vi "LET Transfer v1.vi"() -> ()   [LabVIEW 2010]
doc: "Cont(inuous) Acq(uire) & Chart (hw timed) demonstrates the hardware timed, non-buffered technique of data acquisition. The scan clock on the board controls acquisition timing. Acquired scans are read directly from the device's FIFO using AI Single Scan. \n\nThe acquisition is configured with no buffer, and the on-board scan clock started at the selected scan rate. In the first loop iteration, the newest (most recent) scan is read from the FIFO. In each subsequent loop iteration AI Single Scan is called to read the oldest scan from the FIFO. Then if a scan is missed because the acquisition does not keep up, an error message will be displayed, and the acquisition stopped. Each scan is plotted on the chart after it is read. \n\nA common reason to use non-buffered acquisition is that some kind of processing needs to be done for each data point. You will probably want to add more functions to the diagram to customize this VI for your application. The acquisition rate you can achieve depends on how much processing and display the VI must do. This VI calls a subVI named My Single-Scan Processing. Add whatever processing you need to this subVI, or replace it with one of your own. The data processing subVI also demonstrates how to use error clusters in your own subVIs, so they can be included in the error data flow chain.\n\nBefore running this VI, set the values of the controls on the front panel. Select Show Help Window from the Help menu to see a description of each control. If the values you select for all the controls are values you will usually use, select Make Current Values Default from the Operate menu and save the VI. Or, you may save individual control's default values by popping up on the control, selecting Data Operations, then selecting Make Current Value Default, and saving the VI."
uses:
  <instrlib>/agilent_b2900_series/Agilent B2900 Series/Public/Configure/Measurement/Configure Measurement (Current).vi
  <instrlib>/agilent_b2900_series/Agilent B2900 Series/Public/Configure/Measurement/Configure Measurement (Voltage).vi
  <vilib>/Utility/file.llb/Write To Spreadsheet File (DBL).vi
  <instrlib>/agilent_b2900_series/Agilent B2900 Series/Agilent B2900 Series.lvlib
panel:
  out "Igs array 2":dbl[][](array[numeric])
  out "Vgs array 2":dbl[][](array[numeric])
  out "Vds array 2":dbl[][](array[numeric])
  out "Corrected PD current array 2":dbl[][](array[numeric])
  out "Ids array 2":dbl[][](array[numeric])
  out "corrected PD current array":dbl[](array[numeric])
  out "Vds array":dbl[](array[numeric])
  out "Ids array":dbl[](array[numeric])
  out "Vgs array":dbl[](array[numeric])
  out "Igs array":dbl[](array[numeric])
  in  "Tab Control":T1(tab)
  in  "keithley address":string="GPIB0::20::INSTR"
  in  "agilent address":refnum<visa-resource-name>="GPIB0::23::INSTR"
  in  "Initial Vgs (V)":sgl format="%.2f"
  in  "Vgs step (V)":sgl=1.0 format="%.2f"
  in  "Vgs delay time (ms)":sgl=10.0 format="%.2f"
  in  "Vgs delay after first value":sgl=10.0 caption="Vgs delay after first value (ms)" format="%.2f"
  in  "Final Vgs(V)":sgl=60.0 format="%.2f"
  in  "light emission ON/OFF":bool=TRUE
  in  "Vds step (V)":sgl=20.0 format="%.2f"
  in  "Final Vds (V)":sgl=60.0 format="%.2f"
  in  "Initial Vds (V)":sgl format="%.2f"
  in  "Vds hold time (ms)":i32=10
  in  "Compliance Voltage (channel 1)":dbl=60.0
  in  "Compliance Current (channel 2)":dbl=0.001
  in  "Compliance Voltage (channel 2)":dbl=60.0
  in  "Compliance Current (channel 1)":dbl=0.0001
  in  "keithley compliance limit":dbl(ring)=0.025 items=["25uA"=2.5e-05, "250uA"=0.00025, "2.5mA"=0.0025, "25mA"=0.025]
  in  "Loop":bool=TRUE
  in  "Tab Control 2":enum32{"log scale", "linear scale"}(tab)
  out "Current Scan log":cluster{dbl[], dbl[]}(graph) caption="Current Scan"
  out "Current Scan log2":cluster{dbl[], dbl[]}(graph) caption="Current Scan"
  out "Current Scan linear":cluster{dbl[], dbl[]}(graph) caption="Current Scan"
  out "Current Scan linear 2":cluster{dbl[], dbl[]}(graph) caption="Current Scan"
  out "Applied Vgs":sgl caption="current VDS (V)" format="%.2f"
  out "Applied Vds":sgl caption="current VDS (V)" format="%.2f"
  out "Measured Ids":dbl format="%.2e"
  out "Measured Vds":dbl
  out "corrected PD current":dbl format="%^.2e"
  out "dark PD current (A)":dbl format="%^.2e"
  out "PD current":dbl format="%^.2e"
  out "Measured Igs":dbl
  out "Measured Vgs":dbl
  out "channel 2 status":bool
  out "channel 1 status":bool
  out "half  points":sgl
  out "Vgs points":sgl
  out "Vds points":sgl
  in  "Tab Control 3":enum32{"Log scale", "Linear scale"}(tab)
  out "?":cluster{dbl[], dbl[]}[](graph)
  out "?":cluster{dbl[], dbl[]}[](graph)
  out "?":cluster{dbl[], dbl[]}[](graph)
  out "?":cluster{dbl[], dbl[]}[](graph)
  in  "error in keithley":errorcluster
  out "keithley address out":refnum<k15>
  out "error out keithley":errorcluster
  out "error out agilent":errorcluster
  out "Agilent address out":refnum<visa-resource-name>
  # "LET Transfer v1"
  # "Gate Setting"
  # "Drain-source Setting"
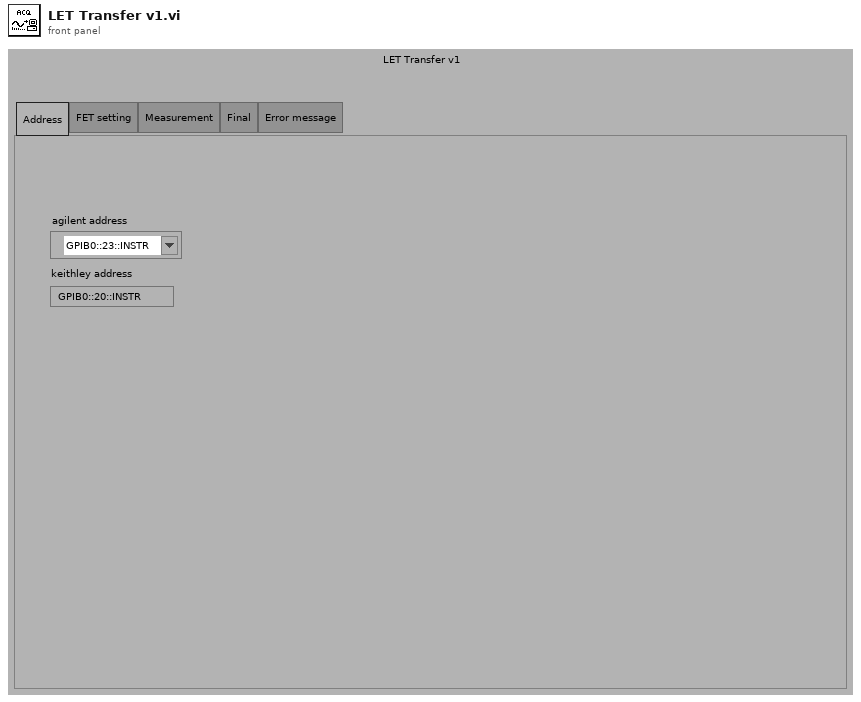
[diagram p1: front panel]
types:
  T1 = enum32{"Address", "FET setting", "Measurement", "Final", "Error message"}
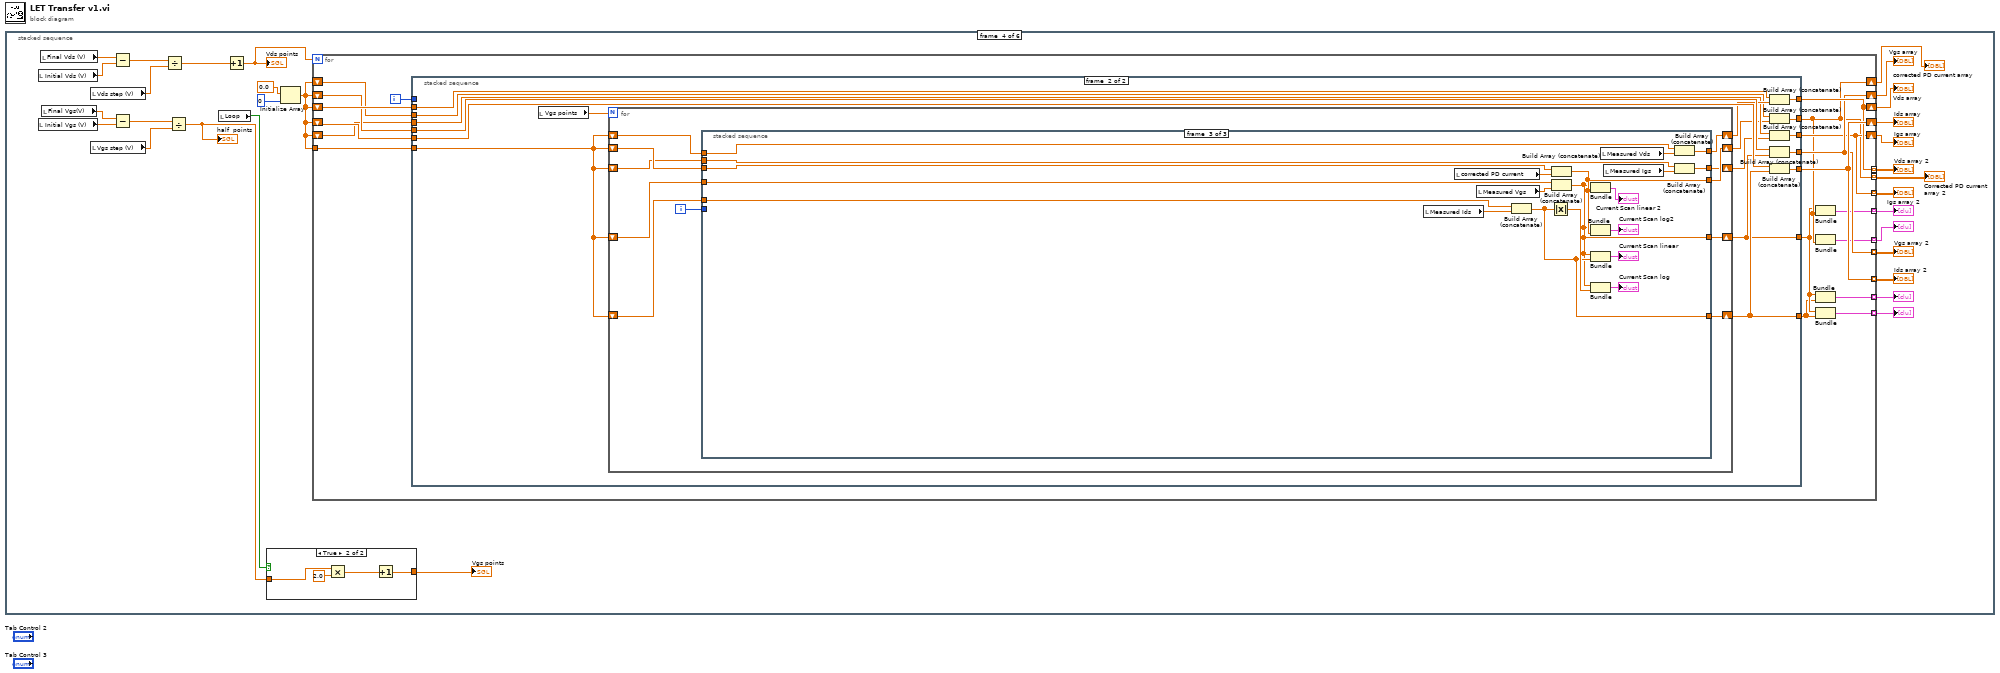
[diagram p0: block diagram]
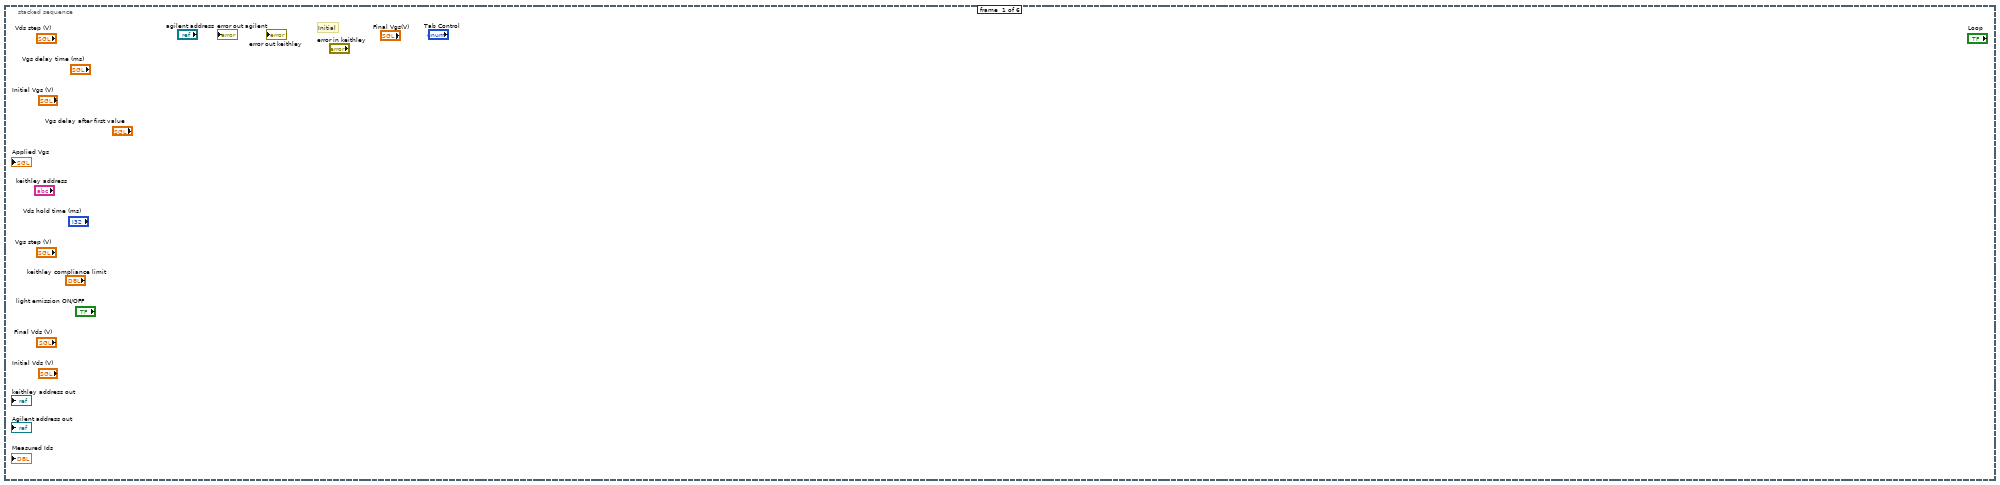
[diagram p2: hidden frame]
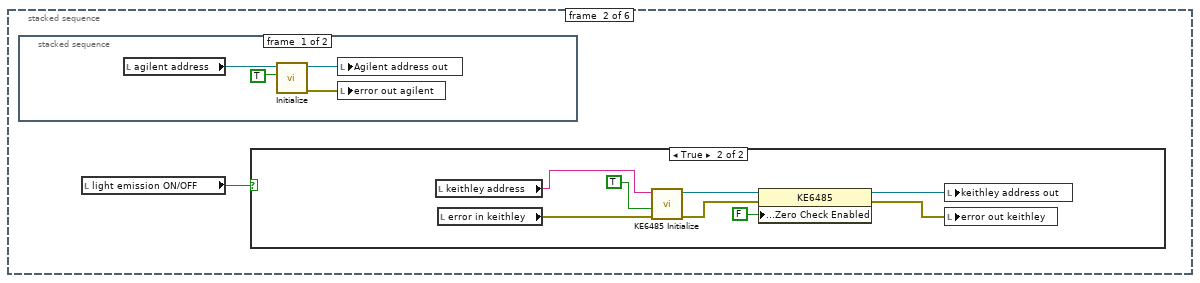
[diagram p3: hidden frame]
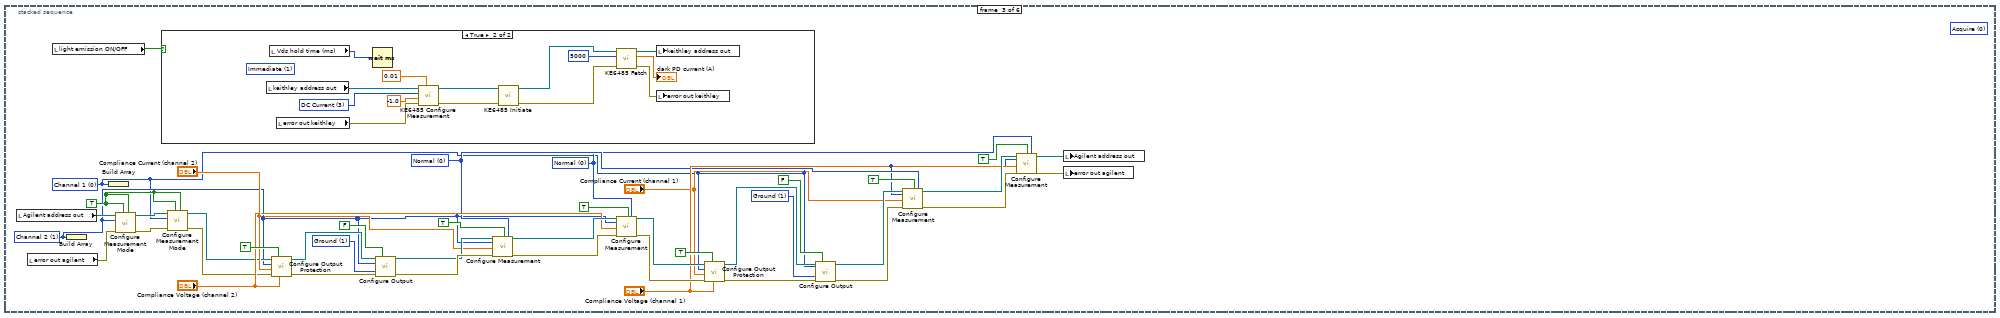
[diagram p6: hidden frame]
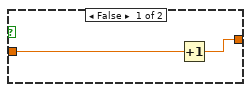
[diagram p8: hidden frame]
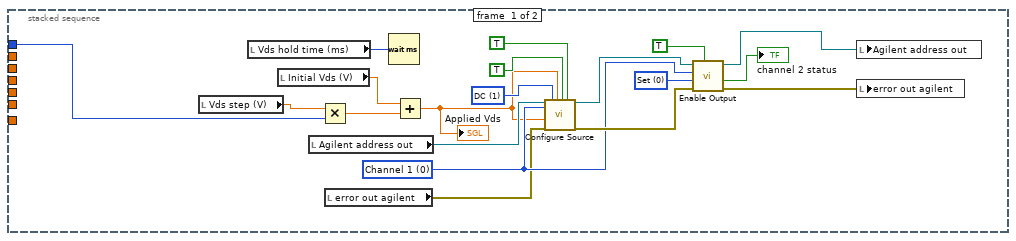
[diagram p9: hidden frame]
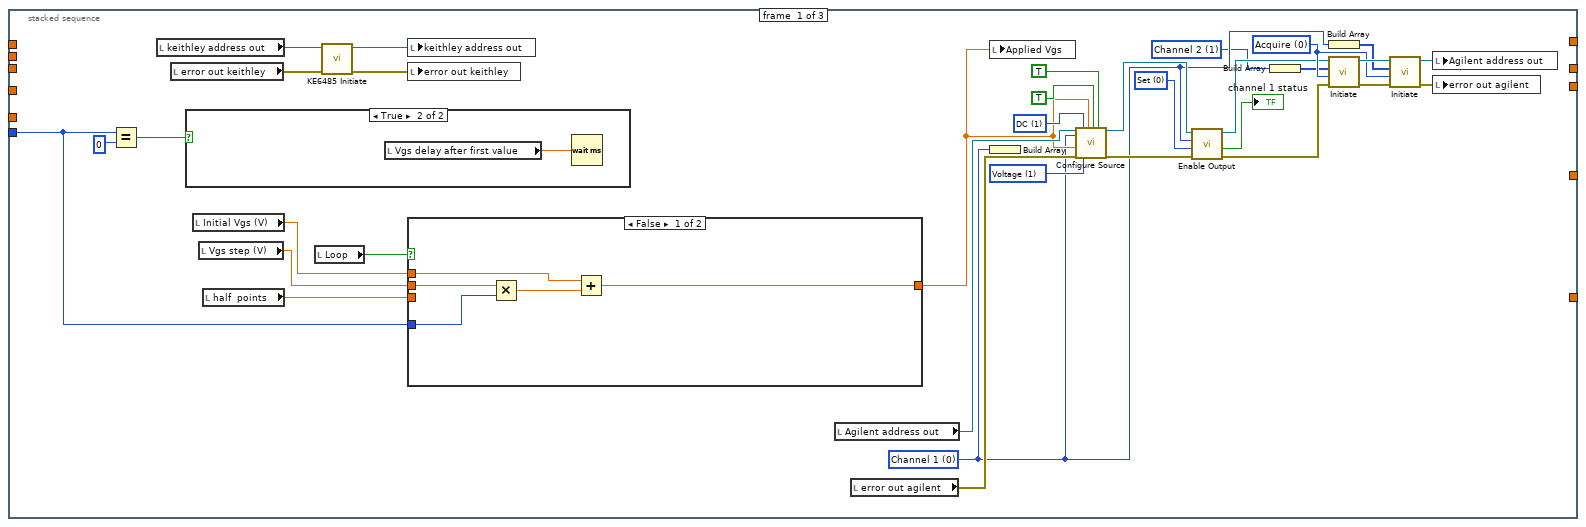
[diagram p10: hidden frame]
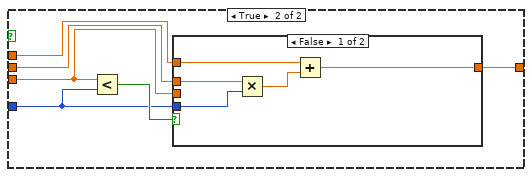
[diagram p11: hidden frame]
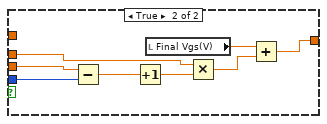
[diagram p12: hidden frame]
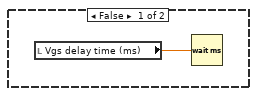
[diagram p13: hidden frame]
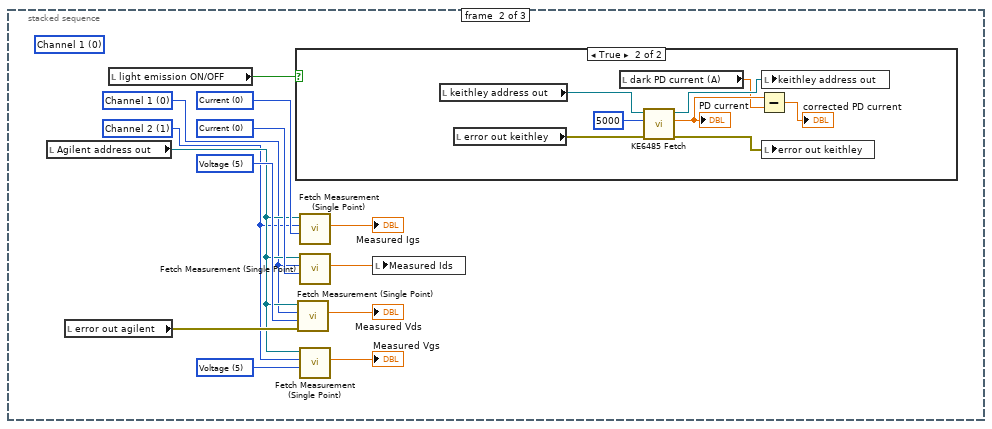
[diagram p14: hidden frame]
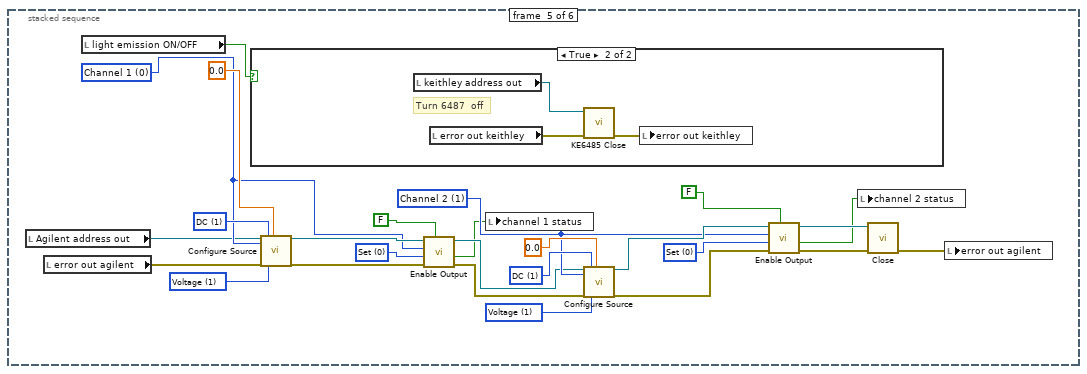
[diagram p16: hidden frame]
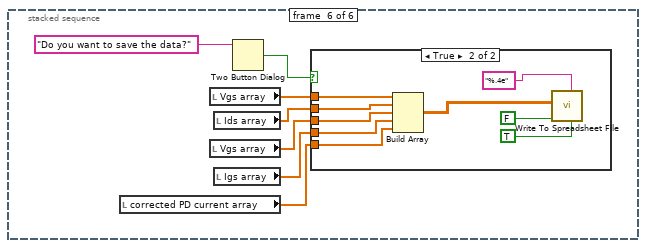
[diagram p18: hidden frame]
diagram:
  n1 = stacked-sequence {
    frame #0 {
      # "Initial"
    }
    frame #1 {
      n2 = stacked-sequence {
        frame #0 {
          n3 = local read "agilent address"() -> (w2:refnum<visa-resource-name>)
          n4 = call <instrlib>:"Initialize.vi"("ID Query (True)"=TRUE, "VISA resource name"=w2) -> ("error out"=w3:errorcluster, "VISA resource name out"=w4:refnum<visa-resource-name>)  [unwired: 8 in]
          n5 = local write "Agilent address out"(w4) -> ()
          n6 = local write "error out agilent"(w3) -> ()
        }
        frame #1 {
        }
      }
      n7 = local read "light emission ON/OFF"() -> (w1:bool)
      n8 = case shown="True" w1 {
        frame False {
        }
        frame True {
          n9 = local read "keithley address"() -> (w12:string)
          n10 = local read "error in keithley"() -> (w13:errorcluster)
          n11 = call <instrlib>:"KE6485 Initialize.vi"("error in (no error)"=w13, "reset device"=TRUE, "resource name"=w12) -> ("error out"=w10:errorcluster, "instrument handle out"=w9:refnum<k15>)  [unwired: 1 in, 6 out]
          n12 = property class="KE6485"(reference=w9, error in=w10, "System Settings:Zero Check Enabled"=FALSE) -> (reference out=w8:refnum<k15>, error out=w7:errorcluster)
          n13 = local write "keithley address out"(w8) -> ()
          n14 = local write "error out keithley"(w7) -> ()
        }
      }
    }
    frame #2 {
      (unwired) 0 items=["Acquire", "Transient", "Both"] ("Device Action (2: Both)")
      w24 = TRUE ("Enable Voltage Measurement (T: Enable)")
      w38 = 1 items=["Float", "Ground"] ("Low Terminal State (1: Ground)")
      w16 = 0 items=["Channel 1", "Channel 2"] ("Channel (0: Channel 1)")
      w26 = 0 items=["Normal", "Resolution", "Speed"] ("Current Auto Range Mode (0: Normal)")
      w48 = 1 items=["Float", "Ground"] ("Low Terminal State (1: Ground)")
      w17 = 1 items=["Channel 1", "Channel 2"] ("Channel (0: Channel 1)")
      w25 = 0 items=["Normal", "Resolution", "Speed"] ("Voltage Auto Range Mode (0: Normal)")
      n15 = local read "Agilent address out"() -> (w19:refnum<visa-resource-name>)
      n16 = local read "error out agilent"() -> (w21:errorcluster)
      n17 = local read "light emission ON/OFF"() -> (w55:bool)
      n18 = Build Array(w17) -> ()  [unwired: 1 out]
      n19 = Build Array(w16) -> ()  [unwired: 1 out]
      n20 = call <instrlib>:"Configure Measurement Mode.vi"("Enable Current Measurement (T: Enable)"=w24, "Enable Voltage Measurement (T: Enable)"=w24, "error in (no error)"=w21, "Channel (0: Channel 1)"=w17, "VISA resource name"=w19) -> ("error out"=w22:errorcluster, "VISA resource name out"=w23:refnum<visa-resource-name>)  [unwired: 5 in]
      n21 = case shown="True" w55 {
        frame False {
        }
        frame True {
          (unwired) 1 items=["Immediate"=1, "Interval"=10, "Trigger Link 1"=1001, "Trigger Link 2"=1002, "Trigger Link 3"=1003, "Trigger Link 4"=1004, "Trigger Link 5"=1005, "Trigger Link 6"=1006] ("sample trigger")
          w67 = 3 items=["DC Volts"=1, "DC Current"=3, "2 Wire Resistance"=5, "Charge"=1004] ("measurement function")
          n22 = local read "keithley address out"() -> (w61:refnum<k15>)
          n23 = local read "Vds hold time (ms)"() -> (w69:i32)
          n24 = local read "error out keithley"() -> (w60:errorcluster)
          n25 = Wait (ms)(milliseconds to wait=w69) -> ()  [unwired: 1 out]
          n26 = call <instrlib>:"KE6485 Configure Measurement.vi"("resolution (absolute)"=0.01, "error in (no error)"=w60, "range"=-1.0, "measurement function"=w67, "instrument handle"=w61) -> ("error out"=w57:errorcluster, "instrument handle out"=w59:refnum<k15>)  [unwired: 5 in]
          n27 = call <instrlib>:"KE6485 Initiate.vi"("error in (no error)"=w57, "instrument handle"=w59) -> ("error out"=w56:errorcluster, "instrument handle out"=w58:refnum<k15>)  [unwired: 8 in]
          n28 = call <instrlib>:"KE6485 Fetch.vi"("error in (no error)"=w56, "maximum time (ms)"=5000, "instrument handle"=w58) -> ("error out"=w64:errorcluster, "reading"=→"dark PD current (A)":dbl, "instrument handle out"=w63:refnum<k15>)  [unwired: 6 in]
          n29 = local write "keithley address out"(w63) -> ()
          n30 = local write "error out keithley"(w64) -> ()
        }
      }
      n31 = call <instrlib>:"Configure Measurement Mode.vi"("Enable Current Measurement (T: Enable)"=w24, "Enable Voltage Measurement (T: Enable)"=w24, "error in (no error)"=w22, "Channel (0: Channel 1)"=w16, "VISA resource name"=w23) -> ("error out"=w20:errorcluster, "VISA resource name out"=w18:refnum<visa-resource-name>)  [unwired: 5 in]
      n32 = call <instrlib>:"Configure Output Protection.vi"("Compliance Voltage (2 V)"="Compliance Voltage (channel 2)", "Enable Output Protection (T: Enable)"=TRUE, "error in (no error)"=w20, "Compliance Current (0.0001 A)"="Compliance Current (channel 2)", "Channel (0: Channel 1)"=w17, "VISA resource name"=w18) -> ("error out"=w50:errorcluster, "VISA resource name out"=w49:refnum<visa-resource-name>)  [unwired: 4 in]
      n33 = call <instrlib>:"Configure Output.vi"("VISA resource name"=w49, "Auto Output-Off (F: Disable)"=FALSE, "Channel (0: Channel 1)"=w17, "Low Terminal State (1: Ground)"=w48, "error in (no error)"=w50) -> ("VISA resource name out"=w46:refnum<visa-resource-name>, "error out"=w47:errorcluster)  [unwired: 9 in]
      n34 = call-poly <instrlib>:"Configure Measurement.vi"("VISA resource name"=w46, "Channel (0: Channel 1)"=w17, "Current Range (0.0001 A)"="Compliance Current (channel 2)", "error in (no error)"=w47, "Current Auto Range (T: Enable)"=TRUE, "Current Auto Range Mode (0: Normal)"=w26) -> ("VISA resource name out"=w54:refnum<visa-resource-name>, "error out"=w53:errorcluster)  [unwired: 12 in]
      n35 = call-poly <instrlib>:"Configure Measurement.vi"("VISA resource name"=w54, "Channel (0: Channel 1)"=w17, "Voltage Range (2 V)"="Compliance Voltage (channel 2)", "error in (no error)"=w53, "Voltage Auto Range (T: Enable)"=TRUE, "Voltage Auto Range Mode (0: Normal)"=w25) -> ("VISA resource name out"=w34:refnum<visa-resource-name>, "error out"=w33:errorcluster)  [unwired: 12 in]
      n36 = call <instrlib>:"Configure Output Protection.vi"("Compliance Voltage (2 V)"="Compliance Voltage (channel 1)", "Enable Output Protection (T: Enable)"=TRUE, "error in (no error)"=w33, "Compliance Current (0.0001 A)"="Compliance Current (channel 1)", "Channel (0: Channel 1)"=w16, "VISA resource name"=w34) -> ("error out"=w40:errorcluster, "VISA resource name out"=w39:refnum<visa-resource-name>)  [unwired: 4 in]
      n37 = call <instrlib>:"Configure Output.vi"("VISA resource name"=w39, "Auto Output-Off (F: Disable)"=FALSE, "Channel (0: Channel 1)"=w16, "Low Terminal State (1: Ground)"=w38, "error in (no error)"=w40) -> ("VISA resource name out"=w36:refnum<visa-resource-name>, "error out"=w37:errorcluster)  [unwired: 9 in]
      n38 = call-poly <instrlib>:"Configure Measurement.vi"("VISA resource name"=w36, "Channel (0: Channel 1)"=w16, "Current Range (0.0001 A)"="Compliance Current (channel 1)", "error in (no error)"=w37, "Current Auto Range (T: Enable)"=TRUE, "Current Auto Range Mode (0: Normal)"=w26) -> ("VISA resource name out"=w44:refnum<visa-resource-name>, "error out"=w43:errorcluster)  [unwired: 12 in]
      n39 = call-poly <instrlib>:"Configure Measurement.vi"("VISA resource name"=w44, "Channel (0: Channel 1)"=w16, "Voltage Range (2 V)"="Compliance Voltage (channel 1)", "error in (no error)"=w43, "Voltage Auto Range (T: Enable)"=TRUE, "Voltage Auto Range Mode (0: Normal)"=w25) -> ("VISA resource name out"=w15:refnum<visa-resource-name>, "error out"=w14:errorcluster)  [unwired: 12 in]
      n40 = local write "Agilent address out"(w15) -> ()
      n41 = local write "error out agilent"(w14) -> ()
    }
    frame #3 {
      n42 = local read "Initial Vds (V)"() -> (w88:sgl)
      n43 = local read "Initial Vgs (V)"() -> (w91:sgl)
      n44 = local read "Final Vds (V)"() -> (w87:sgl)
      n45 = local read "Final Vgs(V)"() -> (w90:sgl)
      n46 = local read "Vds step (V)"() -> (w89:sgl)
      n47 = local read "Vgs step (V)"() -> (w92:sgl)
      n48 = Subtract(x=w87, y=w88) -> (x-y=w85:sgl)
      n49 = Subtract(x=w90, y=w91) -> (x-y=w99:sgl)
      n50 = Divide(x=w85, y=w89) -> (x/y=w86:sgl)
      n51 = Divide(x=w99, y=w92) -> (x/y=w81:sgl)
      "half  points" <- w81
      n52 = local read "Loop"() -> (w82:bool)
      n53 = Increment(x=w86) -> (x+1=w84:sgl)
      "Vds points" <- w84
      n54 = case shown="True" w82 {
        tunnel: w81 -> [w101 w105]
        tunnel: [w100 w103] -> w83
        frame False {
          n55 = Increment(x=w101) -> (x+1=w100:sgl)
        }
        frame True {
          n56 = Multiply(x=w105, y=sgl 2.0) -> (x*y=w102:sgl)
          n57 = Increment(x=w102) -> (x+1=w103:sgl)
        }
      }
      "Vgs points" <- w83
      n58 = Initialize Array(0.0, 0) -> (w78:dbl[])
      n59 = for {
        N: w84 -> [_]
        shift-right: [w114] -> w95
        shift-left: w78 -> [w122]
        shift-right: [w115] -> w96
        shift-left: w78 -> [w121]
        shift-right: [w113] -> w94
        shift-left: w78 -> [w120]
        tunnel: [w119] -> w93 mode=indexing
        shift-right: [w112] -> w80
        shift-left: w78 -> [w118]
        shift-right: [w110] -> w79
        shift-left: w78 -> [w117]
        tunnel: w78 -> [w116]
        tunnel: [w115] -> w77 mode=indexing
        tunnel: [w110] -> w76 mode=indexing
        tunnel: [w114] -> w75 mode=indexing
        tunnel: [w113] -> w74 mode=indexing
        tunnel: [w112] -> w73 mode=indexing
        tunnel: [w111] -> w72 mode=indexing
        tunnel: [w109] -> w71 mode=indexing
        tunnel: [w106] -> w70 mode=indexing
        i -> [w123]
        n60 = stacked-sequence {
          tunnel: w123 -> [w138 _]
          tunnel: w122 -> [_ w159]
          tunnel: w121 -> [_ w158]
          tunnel: [_ w154] -> w114
          tunnel: [_ w157] -> w115
          tunnel: w120 -> [_ w156]
          tunnel: [_ w155] -> w113
          tunnel: [_ w143] -> w108
          tunnel: [_ w152] -> w107
          tunnel: w118 -> [_ w151]
          tunnel: [_ w150] -> w112
          tunnel: [_ w148] -> w110
          tunnel: w117 -> [_ w146]
          tunnel: w116 -> [_ w144]
          frame #0 {
            w131 = 0 items=["Set", "Get"] ("Operation (0: Set)")
            w132 = 0 items=["Channel 1", "Channel 2"] ("Channel (0: Channel 1)")
            w135 = 1 items=["Pulse", "DC"] ("Source Shape (1: DC)")
            n61 = local read "Vds step (V)"() -> (w142:sgl)
            n62 = local read "Vds hold time (ms)"() -> (w140:i32)
            n63 = local read "Initial Vds (V)"() -> (w141:sgl)
            n64 = local read "Agilent address out"() -> (w128:refnum<visa-resource-name>)
            n65 = Multiply(x=w142, y=w138) -> (x*y=w139:sgl)
            n66 = local read "error out agilent"() -> (w127:errorcluster)
            n67 = Wait (ms)(milliseconds to wait=w140) -> ()  [unwired: 1 out]
            n68 = Add(x=w141, y=w139) -> (x+y=w124:sgl)
            "Applied Vds" <- w124
            n69 = call <instrlib>:"Configure Source.vi"("VISA resource name"=w128, "Channel (0: Channel 1)"=w132, "Source Range (2)"=w124, "error in (no error)"=w127, "Source Shape (1: DC)"=w135, "Output Level (0)"=w124, "Source Auto Range (T: Enable)"=TRUE, "Enable Continuous Output (T: Enable)"=TRUE) -> ("VISA resource name out"=w137:refnum<visa-resource-name>, "error out"=w136:errorcluster)  [unwired: 10 in]
            n70 = call <instrlib>:"Enable Output.vi"("Enable Output (T: Enable)"=TRUE, "error in (no error)"=w136, "Operation (0: Set)"=w131, "Channel (0: Channel 1)"=w132, "VISA resource name"=w137) -> ("error out"=w126:errorcluster, "Output Enabled?"=→"channel 2 status":bool, "VISA resource name out"=w125:refnum<visa-resource-name>)  [unwired: 4 in]
            n71 = local write "Agilent address out"(w125) -> ()
            n72 = local write "error out agilent"(w126) -> ()
          }
          frame #1 {
            n73 = local read "Vgs points"() -> (w145:sgl)
            n74 = for {
              N: w145 -> [_]
              shift-right: [w161] -> w152
              shift-left: w144 -> [w160]
              shift-right: [w163] -> w153
              shift-left: w144 -> [w162]
              shift-right: [w167] -> w143
              shift-left: w144 -> [w166]
              shift-right: [w165] -> w149
              shift-left: w144 -> [w164]
              shift-right: [w168] -> w147
              shift-left: w144 -> [w169]
              i -> [w170]
              n75 = stacked-sequence {
                tunnel: w170 -> [w190 _ _]
                tunnel: w169 -> [_ _ w269]
                tunnel: [_ _ w254] -> w168
                tunnel: [_ _ w251] -> w167
                tunnel: w166 -> [_ _ w267]
                tunnel: [_ _ w253] -> w165
                tunnel: w164 -> [_ _ w265]
                tunnel: [_ _ w258] -> w163
                tunnel: w162 -> [_ _ w262]
                tunnel: [_ _ w252] -> w161
                tunnel: w160 -> [_ _ w260]
                frame #0 {
                  w183 = 0 items=["Acquire", "Transient", "Both"] ("Device Action (2: Both)")
                  w175 = 1 items=["Channel 1", "Channel 2"] ("Channel (0: Channel 1)")
                  w192 = 1 items=["Current", "Voltage"] ("Source Mode (1: Voltage)")
                  w195 = 1 items=["Pulse", "DC"] ("Source Shape (1: DC)")
                  w176 = 0 items=["Channel 1", "Channel 2"] ("Channel (0: Channel 1)")
                  w199 = 0 items=["Set", "Get"] ("Operation (0: Set)")
                  n76 = Equal?(x=w190, y=0) -> (x = y?=w202:bool)
                  n77 = local read "keithley address out"() -> (w172:refnum<k15>)
                  n78 = local read "error out keithley"() -> (w171:errorcluster)
                  n79 = case shown="True" w202 {
                    frame False {
                      n80 = local read "Vgs delay time (ms)"() -> (w228:sgl)
                      n81 = Wait (ms)(milliseconds to wait=w228) -> ()  [unwired: 1 out]
                    }
                    frame True {
                      n82 = local read "Vgs delay after first value"() -> (w229:sgl)
                      n83 = Wait (ms)(milliseconds to wait=w229) -> ()  [unwired: 1 out]
                    }
                  }
                  n84 = local read "Initial Vgs (V)"() -> (w191:sgl)
                  n85 = local read "Vgs step (V)"() -> (w189:sgl)
                  n86 = local read "half  points"() -> (w187:sgl)
                  n87 = local read "Loop"() -> (w188:bool)
                  n88 = call <instrlib>:"KE6485 Initiate.vi"("error in (no error)"=w171, "instrument handle"=w172) -> ("error out"=w174:errorcluster, "instrument handle out"=w173:refnum<k15>)  [unwired: 8 in]
                  n89 = local write "keithley address out"(w173) -> ()
                  n90 = local write "error out keithley"(w174) -> ()
                  n91 = case shown="False" w188 {
                    tunnel: [w207 w213] -> w186
                    tunnel: w190 -> [w206 w210]
                    tunnel: w191 -> [w205 w212]
                    tunnel: w189 -> [w204 w211]
                    tunnel: w187 -> [_ w209]
                    frame False {
                      n92 = Multiply(x=w204, y=w206) -> (x*y=w208:sgl)
                      n93 = Add(x=w205, y=w208) -> (x+y=w207:sgl)
                    }
                    frame True {
                      n94 = Less?(x=w209, y=w210) -> (x < y?=w214:bool)
                      n95 = case shown="False" w214 {
                        tunnel: [w218 w227] -> w213
                        tunnel: w212 -> [w217 _]
                        tunnel: w210 -> [w216 w224]
                        tunnel: w211 -> [w215 w225]
                        tunnel: w209 -> [_ w223]
                        frame False {
                          n96 = Multiply(x=w215, y=w216) -> (x*y=w219:sgl)
                          n97 = Add(x=w217, y=w219) -> (x+y=w218:sgl)
                        }
                        frame True {
                          n98 = Subtract(x=w223, y=w224) -> (x-y=w221:sgl)
                          n99 = Increment(x=w221) -> (x+1=w220:sgl)
                          n100 = local read "Final Vgs(V)"() -> (w222:sgl)
                          n101 = Multiply(x=w225, y=w220) -> (x*y=w226:sgl)
                          n102 = Add(x=w222, y=w226) -> (x+y=w227:sgl)
                        }
                      }
                    }
                  }
                  n103 = local read "Agilent address out"() -> (w197:refnum<visa-resource-name>)
                  n104 = local read "error out agilent"() -> (w196:errorcluster)
                  n105 = local write "Applied Vgs"(w186) -> ()
                  n106 = Build Array(w176) -> ()  [unwired: 1 out]
                  n107 = call <instrlib>:"Configure Source.vi"("VISA resource name"=w197, "Channel (0: Channel 1)"=w176, "Source Range (2)"=w186, "error in (no error)"=w196, "Source Shape (1: DC)"=w195, "Source Mode (1: Voltage)"=w192, "Output Level (0)"=w186, "Source Auto Range (T: Enable)"=TRUE, "Enable Continuous Output (T: Enable)"=TRUE) -> ("VISA resource name out"=w201:refnum<visa-resource-name>, "error out"=w200:errorcluster)  [unwired: 9 in]
                  n108 = call <instrlib>:"Enable Output.vi"("error in (no error)"=w200, "Operation (0: Set)"=w199, "Channel (0: Channel 1)"=w176, "VISA resource name"=w201) -> ("error out"=w179:errorcluster, "Output Enabled?"=→"channel 1 status":bool, "VISA resource name out"=w180:refnum<visa-resource-name>)  [unwired: 5 in]
                  n109 = Build Array(w175) -> (w182:i32[])
                  n110 = Build Array(w176) -> (w181:i32[])
                  n111 = call <instrlib>:"Initiate.vi"("error in (no error)"=w179, "Device Action (2: Both)"=w183, "Channel List ({Channel1})"=w182, "VISA resource name"=w180) -> ("error out"=w185:errorcluster, "VISA resource name out"=w184:refnum<visa-resource-name>)  [unwired: 6 in]
                  n112 = call <instrlib>:"Initiate.vi"("error in (no error)"=w185, "Device Action (2: Both)"=w183, "Channel List ({Channel1})"=w181, "VISA resource name"=w184) -> ("error out"=w178:errorcluster, "VISA resource name out"=w177:refnum<visa-resource-name>)  [unwired: 6 in]
                  n113 = local write "Agilent address out"(w177) -> ()
                  n114 = local write "error out agilent"(w178) -> ()
                }
                frame #1 {
                  w231 = 1 items=["Channel 1", "Channel 2"] ("Channel (0: Channel 1)")
                  w232 = 0 items=["Channel 1", "Channel 2"] ("Channel (0: Channel 1)")
                  w237 = 0 items=["Current", "Resistance", "Source Output Setting", "Status", "Time", "Voltage"] ("Data Mode (5: Voltage)")
                  w238 = 5 items=["Current", "Resistance", "Source Output Setting", "Status", "Time", "Voltage"] ("Data Mode (5: Voltage)")
                  w240 = 0 items=["Current", "Resistance", "Source Output Setting", "Status", "Time", "Voltage"] ("Data Mode (5: Voltage)")
                  (unwired) 0 items=["Channel 1", "Channel 2"] ("Channel (0: Channel 1)")
                  w242 = 5 items=["Current", "Resistance", "Source Output Setting", "Status", "Time", "Voltage"] ("Data Mode (5: Voltage)")
                  n115 = local read "Agilent address out"() -> (w233:refnum<visa-resource-name>)
                  n116 = local read "error out agilent"() -> (w234:errorcluster)
                  n117 = local read "light emission ON/OFF"() -> (w230:bool)
                  n118 = case shown="True" w230 {
                    frame False {
                    }
                    frame True {
                      n119 = local read "keithley address out"() -> (w244:refnum<k15>)
                      n120 = local read "error out keithley"() -> (w243:errorcluster)
                      n121 = local read "dark PD current (A)"() -> (w245:dbl)
                      n122 = call <instrlib>:"KE6485 Fetch.vi"("error in (no error)"=w243, "maximum time (ms)"=5000, "instrument handle"=w244) -> ("error out"=w249:errorcluster, "reading"=w246:dbl, "instrument handle out"=w248:refnum<k15>)  [unwired: 6 in]
                      "PD current" <- w246
                      n123 = Subtract(x=w246, y=w245) -> (x-y=→"corrected PD current":dbl)
                      n124 = local write "keithley address out"(w248) -> ()
                      n125 = local write "error out keithley"(w249) -> ()
                    }
                  }
                  n126 = call <instrlib>:"Fetch Measurement (Single Point).vi"("error in (no error)"=w234, "Data Mode (5: Voltage)"=w242, "Channel (0: Channel 1)"=w232, "VISA resource name"=w233) -> ("Measurement"=→"Measured Vds":dbl)  [unwired: 5 in, 2 out]
                  n127 = call <instrlib>:"Fetch Measurement (Single Point).vi"("Data Mode (5: Voltage)"=w237, "Channel (0: Channel 1)"=w231, "VISA resource name"=w233) -> ("Measurement"=→"Measured Igs":dbl)  [unwired: 6 in, 2 out]
                  n128 = call <instrlib>:"Fetch Measurement (Single Point).vi"("Data Mode (5: Voltage)"=w240, "Channel (0: Channel 1)"=w232, "VISA resource name"=w233) -> ("Measurement"=w239:dbl)  [unwired: 6 in, 2 out]
                  n129 = call <instrlib>:"Fetch Measurement (Single Point).vi"("Data Mode (5: Voltage)"=w238, "Channel (0: Channel 1)"=w231, "VISA resource name"=w233) -> ("Measurement"=→"Measured Vgs":dbl)  [unwired: 6 in, 2 out]
                  n130 = local write "Measured Ids"(w239) -> ()
                }
                frame #2 {
                  n131 = local read "Measured Ids"() -> (w261:dbl)
                  n132 = local read "corrected PD current"() -> (w270:dbl)
                  n133 = local read "Measured Vgs"() -> (w268:dbl)
                  n134 = Build Array (concatenate)(w260, w261) -> (w252:dbl[])
                  n135 = Absolute Value(x=w252) -> (abs(x)=w257:dbl[])
                  n136 = Build Array (concatenate)(w269, w270) -> (w254:dbl[])
                  n137 = Build Array (concatenate)(w267, w268) -> (w251:dbl[])
                  n138 = Bundle(w251, w254) -> (→"Current Scan linear 2":cluster{dbl[], dbl[]})  [unwired: 1 out]
                  n139 = Bundle(w251, w254) -> (→"Current Scan log2":cluster{dbl[], dbl[]})  [unwired: 1 out]
                  n140 = Bundle(w251, w252) -> (→"Current Scan linear":cluster{dbl[], dbl[]})  [unwired: 1 out]
                  n141 = Bundle(w251, w257) -> (→"Current Scan log":cluster{dbl[], dbl[]})  [unwired: 1 out]
                  n142 = local read "Measured Vds"() -> (w263:dbl)
                  n143 = local read "Measured Igs"() -> (w266:dbl)
                  n144 = Build Array (concatenate)(w262, w263) -> (w258:dbl[])
                  n145 = Build Array (concatenate)(w265, w266) -> (w253:dbl[])
                }
              }
            }
            n146 = Build Array (concatenate)(w159, w153) -> (w154:dbl[])
            n147 = Build Array (concatenate)(w146, w147) -> (w148:dbl[])
            n148 = Build Array (concatenate)(w151, w149) -> (w150:dbl[])
            n149 = Build Array (concatenate)(w156, w143) -> (w155:dbl[])
            n150 = Build Array (concatenate)(w158, w152) -> (w157:dbl[])
          }
        }
        n151 = Bundle(w108, w110) -> (w111:cluster{dbl[], dbl[]})  [unwired: 1 out]
        n152 = Bundle(w108, w110) -> (w109:cluster{dbl[], dbl[]})  [unwired: 1 out]
        n153 = Bundle(w108, w107) -> (w119:cluster{dbl[], dbl[]})  [unwired: 1 out]
        n154 = Bundle(w108, w107) -> (w106:cluster{dbl[], dbl[]})  [unwired: 1 out]
      }
      "?" <- w93
      "Igs array" <- w80
      "Vgs array" <- w94
      "Ids array" <- w96
      "Vds array" <- w95
      "corrected PD current array" <- w79
      "Ids array 2" <- w77
      "Corrected PD current array 2" <- w76
      "Vds array 2" <- w75
      "Vgs array 2" <- w74
      "Igs array 2" <- w73
      "?" <- w72
      "?" <- w70
      "?" <- w71
    }
    frame #4 {
      w281 = 0 items=["Set", "Get"] ("Operation (0: Set)")
      w283 = 1 items=["Current", "Voltage"] ("Source Mode (1: Voltage)")
      w280 = 1 items=["Channel 1", "Channel 2"] ("Channel (0: Channel 1)")
      w284 = 1 items=["Pulse", "DC"] ("Source Shape (1: DC)")
      w289 = 0 items=["Set", "Get"] ("Operation (0: Set)")
      w291 = 1 items=["Current", "Voltage"] ("Source Mode (1: Voltage)")
      w288 = 0 items=["Channel 1", "Channel 2"] ("Channel (0: Channel 1)")
      w292 = 1 items=["Pulse", "DC"] ("Source Shape (1: DC)")
      n155 = local read "Agilent address out"() -> (w272:refnum<visa-resource-name>)
      n156 = local read "error out agilent"() -> (w271:errorcluster)
      n157 = local read "light emission ON/OFF"() -> (w296:bool)
      n158 = case shown="True" w296 {
        frame False {
        }
        frame True {
          # "Turn 6487  off"
          n159 = local read "keithley address out"() -> (w298:refnum<k15>)
          n160 = local read "error out keithley"() -> (w297:errorcluster)
          n161 = call <instrlib>:"KE6485 Close.vi"("error in (no error)"=w297, "instrument handle"=w298) -> ("error out"=w299:errorcluster)  [unwired: 9 out]
          n162 = local write "error out keithley"(w299) -> ()
        }
      }
      n163 = call <instrlib>:"Configure Source.vi"("VISA resource name"=w272, "Channel (0: Channel 1)"=w288, "error in (no error)"=w271, "Source Shape (1: DC)"=w292, "Source Mode (1: Voltage)"=w291, "Output Level (0)"=0.0) -> ("VISA resource name out"=w294:refnum<visa-resource-name>, "error out"=w290:errorcluster)  [unwired: 12 in]
      n164 = call <instrlib>:"Enable Output.vi"("Enable Output (T: Enable)"=FALSE, "error in (no error)"=w290, "Operation (0: Set)"=w289, "Channel (0: Channel 1)"=w288, "VISA resource name"=w294) -> ("error out"=w278:errorcluster, "Output Enabled?"=w274:bool, "VISA resource name out"=w279:refnum<visa-resource-name>)  [unwired: 4 in]
      n165 = local write "channel 1 status"(w274) -> ()
      n166 = call <instrlib>:"Configure Source.vi"("VISA resource name"=w279, "Channel (0: Channel 1)"=w280, "error in (no error)"=w278, "Source Shape (1: DC)"=w284, "Source Mode (1: Voltage)"=w283, "Output Level (0)"=0.0) -> ("VISA resource name out"=w286:refnum<visa-resource-name>, "error out"=w282:errorcluster)  [unwired: 12 in]
      n167 = call <instrlib>:"Enable Output.vi"("Enable Output (T: Enable)"=FALSE, "error in (no error)"=w282, "Operation (0: Set)"=w281, "Channel (0: Channel 1)"=w280, "VISA resource name"=w286) -> ("error out"=w277:errorcluster, "Output Enabled?"=w275:bool, "VISA resource name out"=w276:refnum<visa-resource-name>)  [unwired: 4 in]
      n168 = local write "channel 2 status"(w275) -> ()
      n169 = call <instrlib>:"Close.vi"("error in (no error)"=w277, "VISA resource name"=w276) -> ("error out"=w273:errorcluster)  [unwired: 9 in]
      n170 = local write "error out agilent"(w273) -> ()
    }
    frame #5 {
      n171 = local read "corrected PD current array"() -> (w301:dbl[])
      n172 = local read "Vgs array"() -> (w300:dbl[])
      n173 = local read "Vgs array"() -> (w303:dbl[])
      n174 = local read "Ids array"() -> (w304:dbl[])
      n175 = local read "Igs array"() -> (w302:dbl[])
      n176 = Two Button Dialog(message="Do you want to save the data?") -> (T button?=w305:bool)  [unwired: 2 out]
      n177 = case shown="True" w305 {
        tunnel: w303 -> [_ w312]
        tunnel: w304 -> [_ w311]
        tunnel: w302 -> [_ w308]
        tunnel: w301 -> [_ w307]
        tunnel: w300 -> [_ w310]
        frame False {
        }
        frame True {
          n178 = Build Array(w310, w311, w312, w308, w307) -> (w309:dbl[][])
          n179 = call-poly <vilib>:"Write To Spreadsheet File.vi"("transpose? (no:F)"=TRUE, "format (%.3f)"="%.4e", "append to file? (new file:F)"=FALSE, "2D data"=w309) -> ()  [unwired: 4 in, 1 out]
        }
      }
    }
  }
